vi "Pre-append object type byte.vi"(8 "error in (no error)":errorcluster, 10 "bytes in":u8[](array[numeric]), 11 "Object type":T1) -> (0 "error out (no error)":errorcluster, 3 "encoded bytes":u8[](array[numeric]) format="%x")   [LabVIEW 2020, in "MessagePack.lvlib"]
uses:
  Typedefs/MsgPack Object Types.ctl
  <vilib>/Utility/error.llb/Error Cluster From Error Code.vi
  <vilib>/ErrorRing/Error Ring.xnode
  MessagePack.lvlib
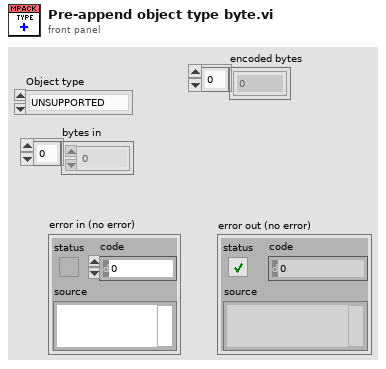
[diagram p1: front panel]
types:
  T1 = typedef "MessagePack.lvlib/MsgPack Object Types.ctl" = enum16{"UNSUPPORTED", "POSINT", "NEGINT", "FIXMAP", "FIXARRAY", "FIXSTR", "NIL", "FALSE", "TRUE", "BIN8", "BIN16", "BIN32", "EXT8", "EXT16", "EXT32", "FLOAT32", "FLOAT64", "UINT8", "UINT16", "UINT32", "UINT64", "INT8", "INT16", "INT32", "INT64", "FIXEXT1", "FIXEXT2", "FIXEXT4", "FIXEXT8", "FIXEXT16", "STR8", "STR16", "STR32", "ARRAY16", "ARRAY32", "MAP16", "MAP32"}
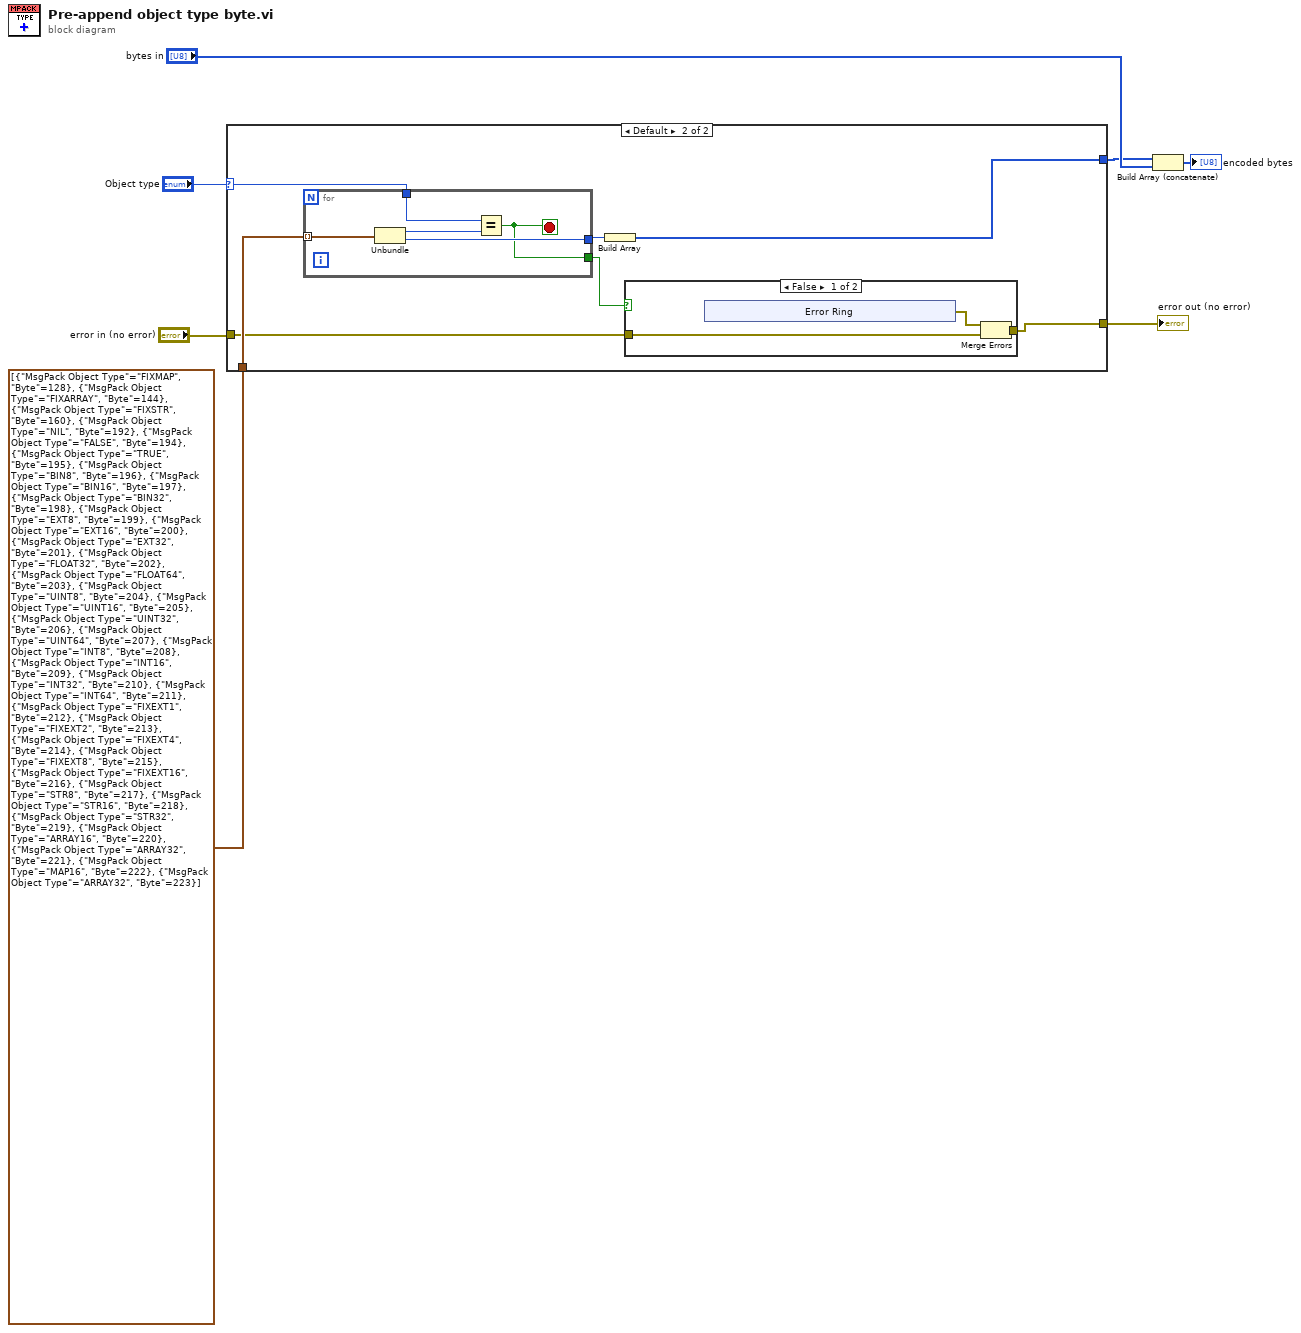
[diagram p0: block diagram]
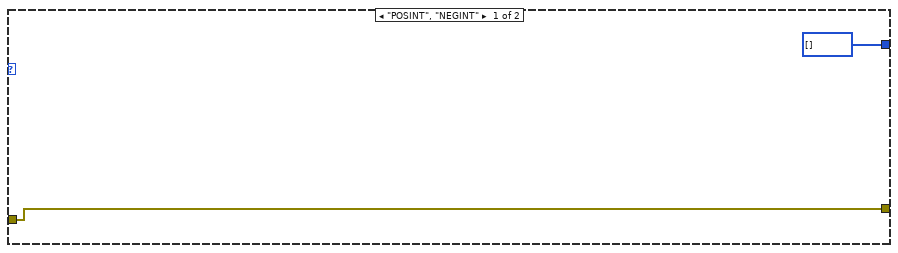
[diagram p2: hidden frame]
diagram:
  n1 = case shown="Default" "Object type" {
    selector: "Object type" -> [_ w15]
    tunnel: cluster{"MsgPack Object Type":T1, "Byte":u8}[] [{"MsgPack Object Type"=enum."FIXMAP", "Byte"=128}, {"MsgPack Object Type"=enum."FIXARRAY", "Byte"=144}, {"MsgPack Object Type"=enum."FIXSTR", "Byte"=160}, {"MsgPack Object Type"=enum."NIL", "Byte"=192}, {"MsgPack Object Type"=enum."FALSE", "Byte"=194}, {"MsgPack Object Type"=enum."TRUE", "Byte"=195}, {"MsgPack Object Type"=enum."BIN8", "Byte"=196}, {"MsgPack Object Type"=enum."BIN16", "Byte"=197}, {"MsgPack Object Type"=enum."BIN32", "Byte"=198}, {"MsgPack Object Type"=enum."EXT8", "Byte"=199}, {"MsgPack Object Type"=enum."EXT16", "Byte"=200}, {"MsgPack Object Type"=enum."EXT32", "Byte"=201}, {"MsgPack Object Type"=enum."FLOAT32", "Byte"=202}, {"MsgPack Object Type"=enum."FLOAT64", "Byte"=203}, {"MsgPack Object Type"=enum."UINT8", "Byte"=204}, {"MsgPack Object Type"=enum."UINT16", "Byte"=205}, {"MsgPack Object Type"=enum."UINT32", "Byte"=206}, {"MsgPack Object Type"=enum."UINT64", "Byte"=207}, {"MsgPack Object Type"=enum."INT8", "Byte"=208}, {"MsgPack Object Type"=enum."INT16", "Byte"=209}, {"MsgPack Object Type"=enum."INT32", "Byte"=210}, {"MsgPack Object Type"=enum."INT64", "Byte"=211}, {"MsgPack Object Type"=enum."FIXEXT1", "Byte"=212}, {"MsgPack Object Type"=enum."FIXEXT2", "Byte"=213}, {"MsgPack Object Type"=enum."FIXEXT4", "Byte"=214}, {"MsgPack Object Type"=enum."FIXEXT8", "Byte"=215}, {"MsgPack Object Type"=enum."FIXEXT16", "Byte"=216}, {"MsgPack Object Type"=enum."STR8", "Byte"=217}, {"MsgPack Object Type"=enum."STR16", "Byte"=218}, {"MsgPack Object Type"=enum."STR32", "Byte"=219}, {"MsgPack Object Type"=enum."ARRAY16", "Byte"=220}, {"MsgPack Object Type"=enum."ARRAY32", "Byte"=221}, {"MsgPack Object Type"=enum."MAP16", "Byte"=222}, {"MsgPack Object Type"=enum."ARRAY32", "Byte"=223}] ("Enum") -> [_ w16]
    tunnel: [u8[] [] ("array") w14] -> w3
    tunnel: "error in (no error)" -> [w8 w11]
    tunnel: [w8 w10] -> w1
    frame "POSINT", "NEGINT" {
    }
    frame Default {
      n2 = for {
        tunnel: w16 -> [w29] mode=indexing
        tunnel: w15 -> [w27]
        tunnel: [w26] -> w13
        tunnel: [w25] -> w12
        stop <- w25 stop-if-true
        n3 = Unbundle(w29) -> ("MsgPack Object Type"=w28:T1, "Byte"=w26:u8)
        n4 = Equal?(x=w27, y=w28) -> (x = y?=w25:bool)
      }
      n5 = Build Array(w13) -> (w14:u8[])
      n6 = case shown="False" w12 {
        tunnel: w11 -> [w18 w24]
        tunnel: [w17 w24] -> w10
        frame False {
          n7 = xnode "Error Ring"() -> ("error out"=w19:errorcluster)
          n8 = Merge Errors(w19, w18) -> (w17:errorcluster)
        }
        frame True {
        }
      }
    }
  }
  "error out (no error)" <- w1
  n9 = Build Array (concatenate)(w3, "bytes in") -> (→"encoded bytes":u8[])
